vi "Kinematic Check.vi"(2 "Ref_pos":dbl[](array[numeric]), 3 "Selection":u16(ring) items=["Check Stopping", "Check Moving", "Reached Dest."], 4 "Inst_pos":dbl[](array[numeric]), 5 "Vz":dbl, 6 "Vy":dbl, 7 "Vx":dbl) -> (0 "True?":bool, 1 "Vmax":dbl)   [LabVIEW 2012]
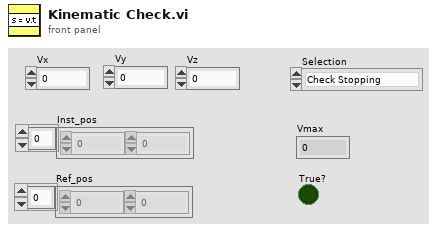
[diagram p1: front panel]
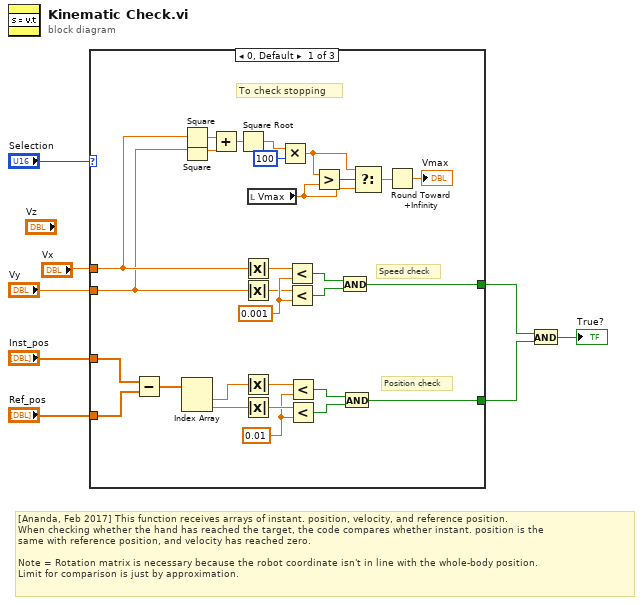
[diagram p0: block diagram]
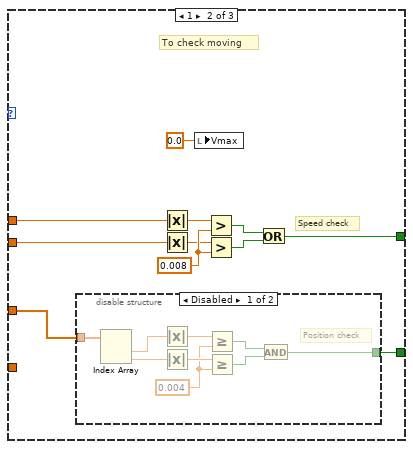
[diagram p2: hidden frame]
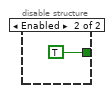
[diagram p3: hidden frame]
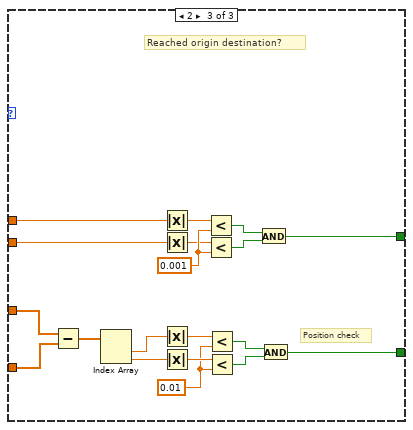
[diagram p4: hidden frame]
diagram:
  # "[Ananda, Feb 2017] This function receives arrays of instant. position, velocity, and reference position.\nWhen checking whether the hand has reached the target, the code compares whether instant. position is the \nsame with reference position, and velocity has reached zero. \n\nNote = Rotation matrix is necessary because the robot coordinate isn't in line with the whole-body position.\nLimit for comparison is just by approximation."
  n1 = case shown="0, Default" "Selection" {
    tunnel: [w24 w41 w72] -> w7
    tunnel: "Inst_pos" -> [w14 w42 w71]
    tunnel: [w32 w43 w63] -> w4
    tunnel: "Ref_pos" -> [w13 _ w70]
    tunnel: "Vy" -> [w9 w39 w60]
    tunnel: "Vx" -> [w10 w38 w59]
    frame 0, Default {
      w25 = 0.01 ("y")
      w35 = 0.001 ("y")
      # "To check stopping"
      # "Position check"
      # "Speed check"
      n2 = Subtract(x=w14, y=w13) -> (x-y=w12:dbl[])
      n3 = Square(x=w10) -> (x^2=w19:dbl)
      n4 = Square(x=w9) -> (x^2=w18:dbl)
      n5 = Index Array(array=w12) -> (element #1=w30:dbl, element #2=w31:dbl)  [unwired: 2 in]
      n6 = Add(x=w19, y=w18) -> (x+y=w20:dbl)
      n7 = Square Root(x=w20) -> (sqrt(x)=w15:dbl)
      n8 = Absolute Value(x=w10) -> (abs(x)=w34:dbl)
      n9 = Absolute Value(x=w9) -> (abs(x)=w33:dbl)
      n10 = Absolute Value(x=w30) -> (abs(x)=w28:dbl)
      n11 = Absolute Value(x=w31) -> (abs(x)=w29:dbl)
      n12 = local read "Vmax"() -> (w17:dbl)
      n13 = Multiply(x=w15, y=u8 100) -> (x*y=w23:dbl)
      n14 = Less?(x=w34, y=w35) -> (x < y?=w36:bool)
      n15 = Less?(x=w33, y=w35) -> (x < y?=w37:bool)
      n16 = Less?(x=w28, y=w25) -> (x < y?=w26:bool)
      n17 = Less?(x=w29, y=w25) -> (x < y?=w27:bool)
      n18 = Greater?(x=w23, y=w17) -> (0:w22:bool)
      n19 = And(x=w36, y=w37) -> (x .and. y?=w32:bool)
      n20 = And(x=w26, y=w27) -> (x .and. y?=w24:bool)
      n21 = Select(t=w23, s=w22, f=w17) -> (s? t:f=w16:dbl)
      n22 = Round Toward +Infinity(x=w16) -> (ceil(x): smallest int >= x=→"Vmax":dbl)
    }
    frame 1 {
      w46 = 0.008 ("y")
      # "To check moving"
      # "Speed check"
      n23 = disable-structure shown="Disabled" {
        disable-tunnel: w42 -> [w50 _]
        disable-tunnel: [w49 TRUE] -> w41
        frame Disabled {
          w51 = 0.004 ("y")
          # "Position check"
          n24 = Index Array(array=w50) -> (element #1=w56:dbl, element #2=w57:dbl)  [unwired: 2 in]
          n25 = Absolute Value(x=w56) -> (abs(x)=w54:dbl)
          n26 = Absolute Value(x=w57) -> (abs(x)=w55:dbl)
          n27 = Greater Or Equal?(x=w54, y=w51) -> (x >= y?=w52:bool)
          n28 = Greater Or Equal?(x=w55, y=w51) -> (x >= y?=w53:bool)
          n29 = And(x=w52, y=w53) -> (x .and. y?=w49:bool)
        }
        frame Enabled {
        }
      }
      n30 = Absolute Value(x=w38) -> (abs(x)=w45:dbl)
      n31 = Absolute Value(x=w39) -> (abs(x)=w44:dbl)
      n32 = local write "Vmax"(0.0 ("Vmax")) -> ()
      n33 = Greater?(x=w45, y=w46) -> (0:w47:bool)
      n34 = Greater?(x=w44, y=w46) -> (0:w48:bool)
      n35 = Or(x=w47, y=w48) -> (x .or. y?=w43:bool)
    }
    frame 2 {
      w66 = 0.001 ("y")
      w62 = 0.01 ("y")
      # "Reached origin destination?"
      # "Position check"
      n36 = Subtract(x=w71, y=w70) -> (x-y=w69:dbl[])
      n37 = Index Array(array=w69) -> (element #1=w61:dbl, element #2=w77:dbl)  [unwired: 2 in]
      n38 = Absolute Value(x=w59) -> (abs(x)=w65:dbl)
      n39 = Absolute Value(x=w60) -> (abs(x)=w64:dbl)
      n40 = Absolute Value(x=w61) -> (abs(x)=w75:dbl)
      n41 = Absolute Value(x=w77) -> (abs(x)=w76:dbl)
      n42 = Less?(x=w65, y=w66) -> (x < y?=w67:bool)
      n43 = Less?(x=w64, y=w66) -> (x < y?=w68:bool)
      n44 = Less?(x=w75, y=w62) -> (x < y?=w73:bool)
      n45 = Less?(x=w76, y=w62) -> (x < y?=w74:bool)
      n46 = And(x=w67, y=w68) -> (x .and. y?=w63:bool)
      n47 = And(x=w73, y=w74) -> (x .and. y?=w72:bool)
    }
  }
  n48 = And(x=w4, y=w7) -> (x .and. y?=→"True?":bool)
